vi "PH_PSDBController.ProcEvents.vi"(0 "i ref in":refnum<vi>, 5 "error in":errorcluster) -> (14 "i ref out":refnum<vi>, 19 "error out":errorcluster)   [LabVIEW 2014, in "PH_PSDBController.lvlib"]
doc: "This method is used to define the events the object will listen to. Add your own events here."
uses:
  PH_PSDBController.lvlib
  CSCore/BaseProcess/BaseProcess.event definition.ctl
  CSCore/CAEObj/CAEObj.event definition.ctl
  CSCore/BaseProcess/BaseProcess.descriptor string definition.ctl
  PH_Common/DIM/PH_DIM.Event Declarer.ctl
  PH_Beamline_Chief/PH_Beamline_Chief.Section.ctl
  CSCore/BaseProcess/BaseProcess.lvlib
  CSCore/CAEObj/CAEObj.lvlib
  PH_Common/PH_Common.lvlib
  PH_Beamline_Chief/PH_Beamline_Chief.lvlib
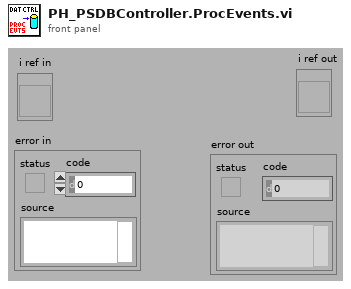
[diagram p1: front panel]
types:
  T1 = typedef "PH_Common.lvlib/PH_DIM.Event Declarer.ctl" = cluster{"Service Name":string, "Selector":string}
  T2 = typedef "BaseProcess.lvlib/BaseProcess.event definition.ctl" = cluster{"CAEEvtDef":T3, "Data Descriptor":T4}
  T3 = typedef "CAEObj.lvlib/CAEObj.event definition.ctl" = cluster{"URL":string, "enable":bool, "ignoreResID":bool}
  T4 = typedef "BaseProcess.lvlib/BaseProcess.descriptor string definition.ctl" = string
  T5 = typedef "PH_Beamline_Chief.lvlib/PH_Beamline_Chief.Section.ctl" = enum16{"None", "YLF", "fs", "fs-YLF", "ns", "PA-Input", "PA-Undelay", "PA-Delay", "PA-before-Bypass", "PA", "PA-Bypass", "PA-Exit", "PA-LL", "LL", "PA-MA", "MA-Exit", "MA-Z6", "Z6", "MA-LB", "LB-TB2", "LB-TB3"}
  T6 = typedef "PH_PSDBController.lvlib/PH_PSDBController.i attribute.ctl" = cluster{"GUI Refs":cluster{"Data Status":refnum<vi>, "Current Shot ID":refnum<vi>, "active Subsystems":refnum<vi>, "Experiment Description":refnum<vi>, "Shot Comment":refnum<vi>, "Experiment":refnum<vi>, "Shottype":refnum<vi>, "Sequencer SM State":refnum<vi>, "Instances with Errors":refnum<vi>}, "Service ID Shot ID":i32, "Service ID wanted Subsystem":i32, "Data Status":T7, "Shotinformation":cluster{"Current Experiment ID":i32, "Current Shot Type":i32, "Current Comment":string}, "Data taking?":bool, "Service ID current Shottype":i32, "Service ID current Experiment":i32, "Service ID currentShot Comment":i32, "Service ID possible Shottypes":i32, "Service ID possible Experiments":i32, "possible Experiments":T8[], "possible Shottypes":T8[], "List":cluster{"Info":cluster{"Instance":string, "Data Status":T7}[], "GUI Ref":refnum<vi>, "Classname":string}[], "Subsystems Off?":cluster{"PHELIX_Beamline_fs_YLF_BL_Status":bool, "PHELIX_Beamline_ns_BL_Status":bool, "PHELIX_Beamline_PA_Input_BL_Status":bool, "PHELIX_Beamline_PA_MA_BL_Status":bool, "PHELIX_Beamline_MA_Z6_BL_Status":bool, "PHELIX_Beamline_MA_LB_BL_Status":bool, "PHELIX_Beamline_PA_LL_BL_Status":bool}, "PSDB Credentials":T9}
  T7 = typedef "PH_PSDBWriter.lvlib/PH_PSDBWriter.Data Status.ctl" = i16
  T8 = typedef "PSDB.lvlib/PSDB_Info.ctl" = cluster{"Name":string, "Description":string, "ID":i32}
  T9 = typedef "PH_Common.lvlib/PH_Connection.PSDB Credentials.ctl" = cluster{"PW":string, "ID":string, "DS":string}
  T10 = cluster{"Info":cluster{"Instance":string, "Data Status":T7}[], "GUI Ref":refnum<vi>, "Classname":string}[]
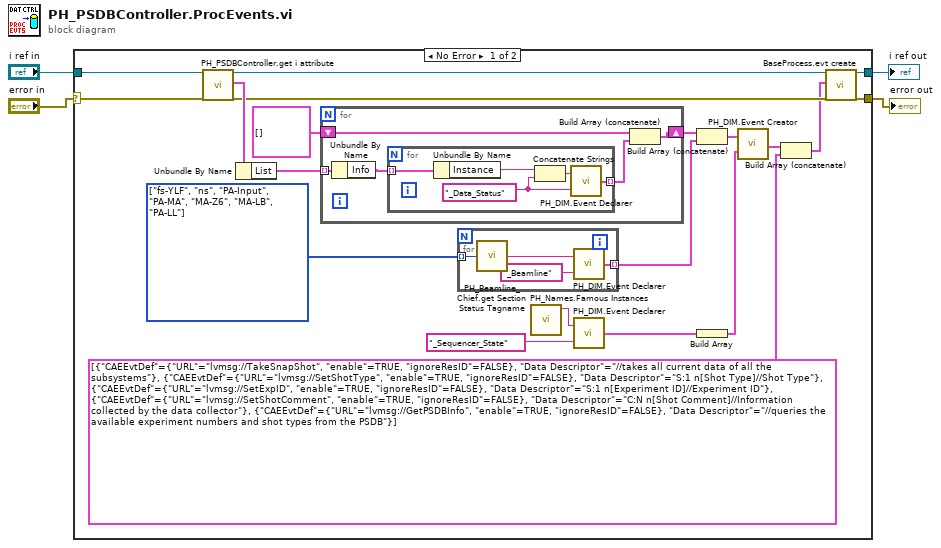
[diagram p0: block diagram]
diagram:
  n1 = case shown="No Error" "error in" {
    selector: "error in" -> [w5 w40]
    tunnel: "i ref in" -> [w6 w39]
    tunnel: [w24 w40] -> w3
    tunnel: [w23 w39] -> w2
    frame No Error {
      w8 = T5[] [enum."fs-YLF", enum."ns", enum."PA-Input", enum."PA-MA", enum."MA-Z6", enum."MA-LB", enum."PA-LL"] items=["None", "YLF", "fs", "fs-YLF", "ns", "PA-Input", "PA-Undelay", "PA-Delay", "PA-before-Bypass", "PA", "PA-Bypass", "PA-Exit", "PA-LL", "LL", "PA-MA", "MA-Exit", "MA-Z6", "Z6", "MA-LB", "LB-TB2", "LB-TB3"]
      n2 = call "PH_PSDBController.get i attribute.vi"("i ref in"=w6, "error in (no error)"=w5) -> ("i ref out"=w20:refnum<vi>, "i attribute"=w22:T6, "error out"=w21:errorcluster)  [unwired: 15 in]
      n3 = Unbundle By Name(w22) -> ("List"=w14:T10)
      n4 = for {
        tunnel: w14 -> [w33] mode=indexing
        shift-right: [w30] -> w11
        shift-left: T1[] [] -> [w29]
        n5 = Unbundle By Name(w33) -> ("Info"=w32:cluster{"Instance":string, "Data Status":T7}[])
        n6 = for {
          tunnel: w32 -> [w36] mode=indexing
          tunnel: [w37] -> w31 mode=indexing
          w34 = "_Data_Status" ("string")
          n7 = Unbundle By Name(w36) -> ("Instance"=w35:string)
          n8 = Concatenate Strings(w35, w34) -> (w38:string)
          n9 = call "PH_DIM.Event Declarer.vi"("Selector"=w34, "Service Name"=w38) -> ("declared DIM Event"=w37:T1)
        }
        n10 = Build Array (concatenate)(w29, w31) -> (w30:T1[])
      }
      n11 = for {
        tunnel: [w27] -> w9 mode=indexing
        tunnel: w8 -> [w25] mode=indexing
        n12 = call "PH_Beamline_Chief.get Section Status Tagname.vi"("Beamline Section"=w25) -> ("Section Status Tagname"=w26:string)
        n13 = call "PH_DIM.Event Declarer.vi"("Selector"="_Beamline" ("string"), "Service Name"=w26) -> ("declared DIM Event"=w27:T1)
      }
      n14 = call "PH_Names.Famous Instances.vi"() -> ("Sequencer"=w7:string)  [unwired: 7 in, 3 out]
      n15 = call "PH_DIM.Event Declarer.vi"("Selector"="_Sequencer_State" ("string"), "Service Name"=w7) -> ("declared DIM Event"=w16:T1)
      n16 = Build Array (concatenate)(w11, w9) -> (w10:T1[])
      n17 = Build Array(w16) -> (w15:T1[])
      n18 = call "PH_DIM.Event Creator.vi"("Trendmessage Services"=w10, "SM State Services"=w15) -> ("DIM Service Events"=w18:T2[])  [unwired: 17 in]
      n19 = Build Array (concatenate)(w18, T2[] [{"CAEEvtDef"={"URL"="lvmsg://TakeSnapShot", "enable"=TRUE, "ignoreResID"=FALSE}, "Data Descriptor"="//takes all current data of all the subsystems"}, {"CAEEvtDef"={"URL"="lvmsg://SetShotType", "enable"=TRUE, "ignoreResID"=FALSE}, "Data Descriptor"="S:1 n[Shot Type]//Shot Type"}, {"CAEEvtDef"={"URL"="lvmsg://SetExpID", "enable"=TRUE, "ignoreResID"=FALSE}, "Data Descriptor"="S:1 n[Experiment ID]//Experiment ID"}, {"CAEEvtDef"={"URL"="lvmsg://SetShotComment", "enable"=TRUE, "ignoreResID"=FALSE}, "Data Descriptor"="C:N n[Shot Comment]//Information collected by the data collector"}, {"CAEEvtDef"={"URL"="lvmsg://GetPSDBInfo", "enable"=TRUE, "ignoreResID"=FALSE}, "Data Descriptor"="//queries the available experiment numbers and shot types from the PSDB"}] ("new events(V3.0)")) -> (w17:T2[])
      n20 = call "BaseProcess.evt create.vi"("i ref in"=w20, "newEvents"=w17, "error in (no error)"=w21) -> ("i ref out"=w23:refnum<vi>, "error out"=w24:errorcluster)  [unwired: 13 in, 2 out]
    }
    frame Error {
    }
  }
  "i ref out" <- w2
  "error out" <- w3
